vi "VGS Volume (from RAW).vi"() -> ()   [LabVIEW 2022 SP3, in "LV_VGS.lvlib"]
uses:
  LV_VGS.lvlib
  typedefs/3D Size (I32).ctl
  typedefs/3D Resolution (SGL).ctl
  RemoteControlClient/VGS_RemoteControlClient.lvclass
  Project/VGS_Project.lvclass
  VolumeDescriptor+File/VGS_VolumeDescriptor+File.lvclass
  VolumeDescriptor/VGS_VolumeDescriptor.lvclass
  ManufacturerInfo/VGS_ManufacturerInfo.lvclass
  ComponentInfo/VGS_ComponentInfo.lvclass
panel:
  out "Save Time, ms":u32
  # "Original Volume Example rewritten in LabVIEW"
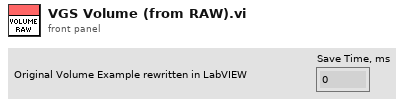
[diagram p1: front panel]
types:
  T1 = typedef "LV_VGS.lvlib/3D Resolution (SGL).ctl" = cluster{"X":sgl, "Y":sgl, "Z":sgl}
  T2 = typedef "LV_VGS.lvlib/3D Size (I32).ctl" = cluster{"X":i32, "Y":i32, "Z":i32}
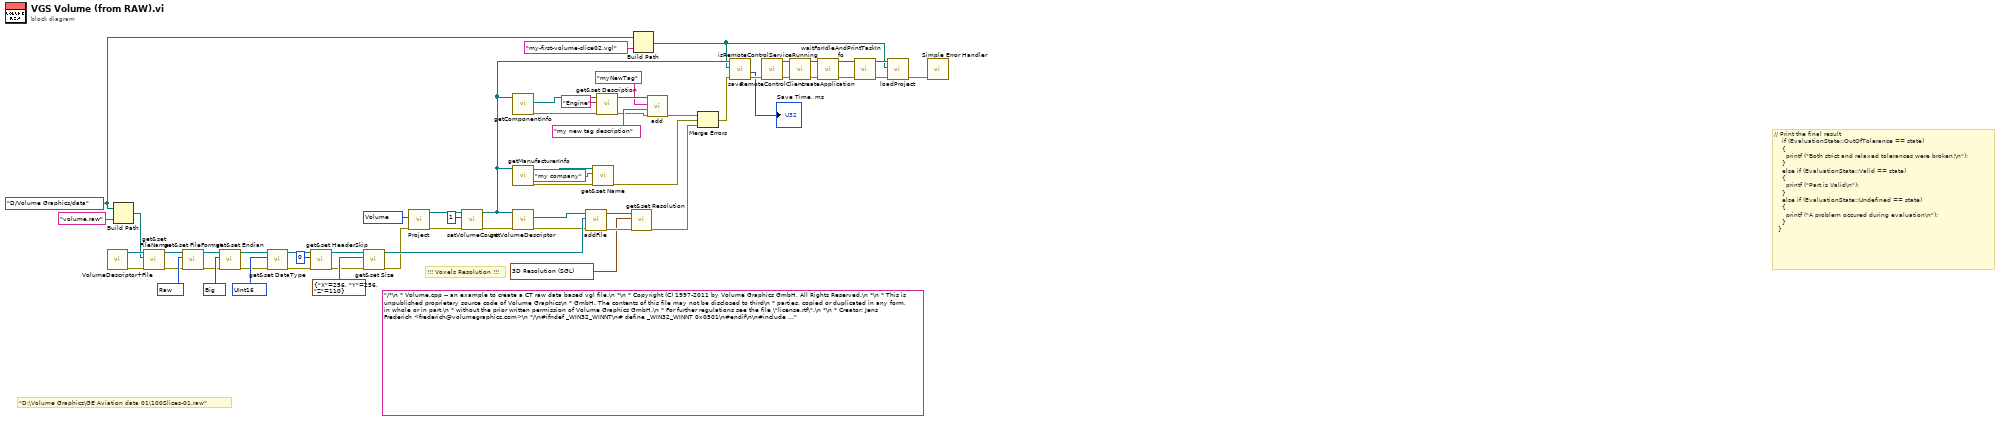
[diagram p0: block diagram]
diagram:
  w5 = 1448153088 items=["Volume"=1448153088, "Reconstruction"=1448153089] ("type")
  w49 = 1448157378 items=["UInt8"=1448157376, "Int8"=1448157377, "UInt16"=1448157378, "Int16"=1448157379, "UInt32"=1448157380, "Int32"=1448157381, "Float"=1448157382, "Rgb8"=1448157383] ("DataType")
  w52 = 1448157441 items=["Little"=1448157440, "Big"=1448157441] ("Endian")
  w55 = 1448157312 items=["Raw"=1448157312, "Gzip"=1448157313, "Tiff"=1448157314, "Jpeg"=1448157315, "Bmp"=1448157316, "Bir"=1448157317, "Toshiba"=1448157318, "Shimadzu"=1448157319, "Pnm"=1448157320, "Jpeg2"=1448157321, "Yxlon"=1448157322, "Hdf"=1448157323, "Dicom"=1448157324, "Imtec"=1448157325, "Aracor"=1448157326, "Fhg"=1448157327] ("FileFormat")
  w7 = path "D:/Volume Graphics/data" ("replacementPattern")
  (unwired) "/*\n * Volume.cpp -- an example to create a CT raw data based vgl file.\n *\n * Copyright (C) 1997-2011 by Volume Graphics GmbH. All Rights Reserved.\n *\n * This is unpublished proprietary source code of Volume Graphics\n * GmbH. The contents of this file may not be disclosed to third\n * parties, copied or duplicated in any form, in whole or in part,\n * without the prior written permission of Volume Graphics GmbH.\n * For further regulations see the file \"license.rtf\".\n *\n * Creator: Jens Frederich <frederich@volumegraphics.com>\n */\n#ifndef _WIN32_WINNT\n# define _WIN32_WINNT 0x0501\n#endif\n\n#include <tchar.h>\n\n#include <vgs.project/project.h>\n\nusing namespace vgs::project;\nusing namespace vgs::project::volume;\n\nint _tmain (int argc, _TCHAR* argv[])\n{\n  Project* p = new Project (Project::Type::Volume);\n  assert (p != NULL);\n\n  // add single raw block file\n  {\n    VolumeDescriptor::File data;\n\n    data.setFileName   (\"D:/Volume Graphics/API TEST/vgs/data/engine.gz\");\n    data.setFileFormat (volume::FileFormat::Gzip);\n    data.setEndian     (volume::Endian::Little);\n    data.setDataType   (DataType::UInt8);\n    data.setHeaderSkip (0);\n    data.setSize       (Vector3<int> (256, 256, 110));\n    \n    p->setVolumeCount (1);\n    VolumeDescriptor* vd = p->getVolumeDescriptor (0);\n    assert (vd != NULL);\n\n    vd->addFile (data);\n  }\n\n  // add some meta data\n  {\n    ManufacturerInfo* mi = p->getManufacturerInfo ();\n    mi->setName (\"My company\");\n\n    ComponentInfo* ci = p->getComponentInfo ();\n    ci->setDescription (\"Engine\");\n\n    // add user defined tag\n    ci->add (\"myNewTag\", \"my new tag description\");\n\n    // add logo and preview\n    //p->setLogo    (\"c:/data/logo.png\");\n    //p->setPreview (\"c:/data/scene_preview.png\");\n  }\n\n  // create VG project\n  {\n    bool ok = true;\n\n    ok = p->save (std::string (\"D:/Volume Graphics/API TEST/vgs/data/my-first-volume1.vgl\"));\n    if (true != ok)\n    {\n      Error::ErrorCode err = Error::getLastError ();\n\t  printf(\"something is wrong, error code = %d\", err);\n      __debugbreak ();\n    }\n  }\n\n  // cleanup\n  if (p != NULL)\n  {\n    delete p;\n  }\n\n  return 0;\n}\n\n"
  # "!!! Voxels Resolution !!!"
  # "\"D:\\Volume Graphics\\GE Aviation data 01\\100Slices-01.raw\""
  # "// Print the final result\n    if (EvaluationState::OutOfTolerance == state)\n    {\n      printf (\"Both strict and relaxed tolerances were broken!\\n\");\n    }\n    else if (EvaluationState::Valid == state)\n    {\n      printf (\"Part is Valid\\n\");\n    }\n    else if (EvaluationState::Undefined == state)\n    {\n      printf (\"A problem occured during evaluation\\n\");\n    }\n  }"
  n1 = call "VolumeDescriptor+File.vi"() -> ("error out"=w57:errorcluster, "VGS_VolumeDescriptor+File out"=w60:refnum<class "VGS_VolumeDescriptor+File.lvclass">)  [unwired: 10 in]
  n2 = Build Path(base path=w7, name or relative path="volume.raw") -> (appended path=w58:path)
  n3 = call "get&set FileName.vi"("error in (no error)"=w57, "FileName"=w58, "VGS_VolumeDescriptor+File in"=w60) -> ("error out"=w54:errorcluster, "VGS_VolumeDescriptor+File out"=w56:refnum<class "VGS_VolumeDescriptor+File.lvclass">)  [unwired: 6 in, 1 out]
  n4 = call "get&set FileFormat.vi"("error in (no error)"=w54, "FileFormat"=w55, "VGS_VolumeDescriptor+File in"=w56) -> ("error out"=w51:errorcluster, "VGS_VolumeDescriptor+File out"=w53:refnum<class "VGS_VolumeDescriptor+File.lvclass">)  [unwired: 6 in, 1 out]
  n5 = call "get&set Endian.vi"("error in (no error)"=w51, "Endian"=w52, "VGS_VolumeDescriptor+File in"=w53) -> ("error out"=w48:errorcluster, "VGS_VolumeDescriptor+File out"=w50:refnum<class "VGS_VolumeDescriptor+File.lvclass">)  [unwired: 6 in, 1 out]
  n6 = call "get&set DataType.vi"("error in (no error)"=w48, "DataType"=w49, "VGS_VolumeDescriptor+File in"=w50) -> ("error out"=w45:errorcluster, "VGS_VolumeDescriptor+File out"=w47:refnum<class "VGS_VolumeDescriptor+File.lvclass">)  [unwired: 6 in, 1 out]
  n7 = call "get&set HeaderSkip.vi"("error in (no error)"=w45, "HeaderSkip"=0, "VGS_VolumeDescriptor+File in"=w47) -> ("error out"=w42:errorcluster, "VGS_VolumeDescriptor+File out"=w44:refnum<class "VGS_VolumeDescriptor+File.lvclass">)  [unwired: 6 in, 1 out]
  n8 = call "get&set Size.vi"("error in (no error)"=w42, "3D Size"=T2 {"X"=256, "Y"=256, "Z"=110}, "VGS_VolumeDescriptor+File in"=w44) -> ("error out"=w9:errorcluster, "VGS_VolumeDescriptor+File out"=w39:refnum<class "VGS_VolumeDescriptor+File.lvclass">)  [unwired: 6 in, 1 out]
  n9 = call "Project.vi"("error in (no error)"=w9, "type"=w5) -> ("error out"=w8:errorcluster, "VGS_Project out"=w41:refnum<class "VGS_Project.lvclass">)  [unwired: 8 in]
  n10 = call "setVolumeCount.vi"("error in (no error)"=w8, "VolumeCount"=u32 1, "VGS_Project in"=w41) -> ("error out"=w37:errorcluster, "VGS_Project out"=w27:refnum<class "VGS_Project.lvclass">)  [unwired: 7 in]
  n11 = call "getComponentInfo.vi"("VGS_Project in"=w27) -> ("error out"=w26:errorcluster, "VGS_ComponentInfo out"=w29:refnum<class "VGS_ComponentInfo.lvclass">)  [unwired: 8 in, 1 out]
  n12 = call "getManufacturerInfo.vi"("VGS_Project in"=w27) -> ("error out"=w24:errorcluster, "LV_VGS.lvlib:VGS_ManufacturerInfo.lvclass"=w28:refnum<class "VGS_ManufacturerInfo.lvclass">)  [unwired: 8 in, 1 out]
  n13 = call "getVolumeDescriptor.vi"("error in (no error)"=w37, "VGS_Project in"=w27) -> ("error out"=w36:errorcluster, "VGS_VolumeDescriptor out"=w38:refnum<class "VGS_VolumeDescriptor.lvclass">)  [unwired: 7 in, 1 out]
  n14 = call "addFile.vi"("error in (no error)"=w36, "LV_VGS.lvlib:VGS_VolumeDescriptor+File.lvclass"=w39, "VGS_VolumeDescriptor in"=w38) -> ("error out"=w4:errorcluster, "VGS_VolumeDescriptor out"=w2:refnum<class "VGS_VolumeDescriptor.lvclass">)  [unwired: 7 in]
  n15 = call "get&set Name.vi"("error in (no error)"=w24, "Name"="my company", "VGS_ManufacturerInfo in"=w28) -> ("error out"=w23:errorcluster)  [unwired: 6 in, 2 out]
  n16 = call "get&set Description.vi"("error in (no error)"=w26, "Description"="Engine", "VGS_ComponentInfo in"=w29) -> ("error out"=w25:errorcluster, "VGS_ComponentInfo out"=w33:refnum<class "VGS_ComponentInfo.lvclass">)  [unwired: 6 in, 1 out]
  n17 = call "get&set Resolution.vi"("error in (no error)"=w4, "3D Resolution"=T1 {"X"=0.0756, "Y"=0.0756, "Z"=0.0756}, "VGS_VolumeDescriptor in"=w2) -> ("error out"=w3:errorcluster)  [unwired: 6 in, 2 out]
  n18 = Build Path(base path=w7, name or relative path="my-first-volume-slice02.vgl") -> (appended path=w10:path)
  n19 = call "add.vi"("error in (no error)"=w25, "description"="my new tag description", "tag"="myNewTag", "VGS_ComponentInfo in"=w33) -> ("error out"=w22:errorcluster)  [unwired: 6 in, 1 out]
  n20 = Merge Errors(w22, w23, w3) -> (w21:errorcluster)
  n21 = call "save.vi"("error in (no error)"=w21, "Path"=w10, "VGS_Project in"=w27) -> ("error out"=w12:errorcluster, "Time, ms"=→"Save Time, ms":u32)  [unwired: 6 in, 1 out]
  n22 = call "RemoteControlClient.vi"("error in (no error)"=w12) -> ("error out"=w14:errorcluster, "VGS_RemoteControlClient out"=w13:refnum<class "VGS_RemoteControlClient.lvclass">)  [unwired: 9 in]
  n23 = call "isRemoteControlServiceRunning.vi"("error in (no error)"=w14, "VGS_RemoteControlClient in"=w13) -> ("error out"=w15:errorcluster, "VGS_RemoteControlClient out"=w16:refnum<class "VGS_RemoteControlClient.lvclass">)  [unwired: 7 in, 1 out]
  n24 = call "createApplication.vi"("error in (no error)"=w15, "VGS_RemoteControlClient in"=w16) -> ("error out"=w17:errorcluster, "VGS_RemoteControlClient out"=w20:refnum<class "VGS_RemoteControlClient.lvclass">)  [unwired: 8 in]
  n25 = call "waitForIdleAndPrintTaskInfo.vi"("error in (no error)"=w17, "VGS_RemoteControlClient in"=w20) -> ("error out"=w18:errorcluster, "VGS_RemoteControlClient out"=w19:refnum<class "VGS_RemoteControlClient.lvclass">)  [unwired: 8 in]
  n26 = call "loadProject.vi"("error in (no error)"=w18, "projectName"=w10, "VGS_RemoteControlClient in"=w19) -> ("error out"=w11:errorcluster)  [unwired: 7 in, 1 out]
  n27 = call <vilib>:"Simple Error Handler.vi"("error in (no error)"=w11) -> ()  [unwired: 4 in, 5 out]
